vi "GDSLvIcon_AnalyseViIcon(ClassFix).vi"(0 "Class Ref":refnum<vi>, 1 "Class Private Data Control VI Ref":refnum<vi>, 3 "DoATextOCR(False)":bool, 5 "error in (no error)":errorcluster) -> (6 "BodyTextColor":u32(colorbox), 7 "Splitter0px":bool, 8 "HeaderTextColor":u32(colorbox), 9 "BodyText(OCR)":string, 10 "FrameColor":u32(colorbox), 11 "HeadText(OCR)":string, 12 "FrameThickness(1)":u32=1, 13 "ValidHeaderIcon":bool, 14 "DefaultIcon":bool, 15 "HeaderIcon":u8[][](array[numeric]) format="%x", 16 "HeaderBkColor":u32(colorbox), 17 "BodyIcon":u8[][](array[numeric]) format="%x", 18 "BodyBkColor":u32(colorbox), 19 "error out":errorcluster)   [LabVIEW 2020]
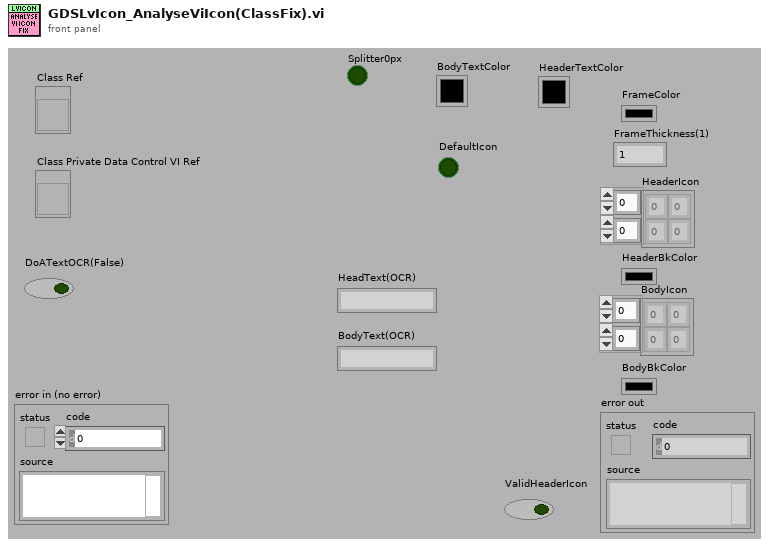
[diagram p1: front panel]
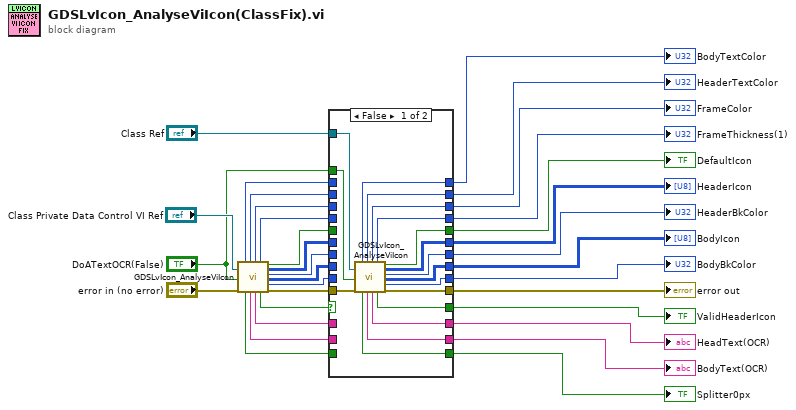
[diagram p0: block diagram]
diagram:
  n1 = call <resource>:"GDSLvIcon_AnalyseViIcon.vi"("ViRef/LvCLassRef/LvLibRef/ViPath/2D_Image"="Class Private Data Control VI Ref", "DoATextOCR(False)"="DoATextOCR(False)", "error in (no error)"="error in (no error)") -> ("BodyTextColor"=w10:u32, "Splitter0px"=w28:bool, "HeaderTextColor"=w12:u32, "BodyText(OCR)"=w27:string, "FrameColor"=w14:u32, "HeadText(OCR)"=w26:string, "FrameThickness(1)"=w16:u32, "ValidHeaderIcon"=w31:bool, "DefaultIcon"=w17:bool, "HeaderIcon"=w22:u8[][], "HeaderBkColor"=w24:u32, "BodyIcon"=w23:u8[][], "BodyBkColor"=w25:u32, "error out"=w5:errorcluster)  [unwired: 3 in]
  n2 = case shown="False" w31 {
    selector: w31 -> [_ w50]
    tunnel: "Class Ref" -> [w49 _]
    tunnel: w28 -> [_ w53]
    tunnel: w27 -> [_ w54]
    tunnel: w26 -> [_ w55]
    tunnel: w25 -> [_ w51]
    tunnel: w24 -> [_ w61]
    tunnel: [w37 w63] -> w20
    tunnel: w23 -> [_ w63]
    tunnel: [w39 w62] -> w21
    tunnel: w22 -> [_ w62]
    tunnel: [w38 w61] -> w19
    tunnel: [w40 w60] -> w18
    tunnel: w17 -> [_ w60]
    tunnel: w16 -> [_ w59]
    tunnel: [w41 w59] -> w15
    tunnel: w14 -> [_ w58]
    tunnel: [w42 w58] -> w13
    tunnel: w12 -> [_ w57]
    tunnel: [w43 w57] -> w11
    tunnel: w10 -> [_ w56]
    tunnel: [w44 w56] -> w9
    tunnel: [w34 w55] -> w8
    tunnel: [w33 w54] -> w7
    tunnel: [w46 w53] -> w6
    tunnel: w5 -> [w48 w52]
    tunnel: [w47 w52] -> w4
    tunnel: "DoATextOCR(False)" -> [w45 _]
    tunnel: [w36 w51] -> w1
    tunnel: [w35 w50] -> w2
    frame False {
      n3 = call <resource>:"GDSLvIcon_AnalyseViIcon.vi"("ViRef/LvCLassRef/LvLibRef/ViPath/2D_Image"=w49, "DoATextOCR(False)"=w45, "error in (no error)"=w48) -> ("BodyTextColor"=w44:u32, "Splitter0px"=w46:bool, "HeaderTextColor"=w43:u32, "BodyText(OCR)"=w33:string, "FrameColor"=w42:u32, "HeadText(OCR)"=w34:string, "FrameThickness(1)"=w41:u32, "ValidHeaderIcon"=w35:bool, "DefaultIcon"=w40:bool, "HeaderIcon"=w39:u8[][], "HeaderBkColor"=w38:u32, "BodyIcon"=w37:u8[][], "BodyBkColor"=w36:u32, "error out"=w47:errorcluster)  [unwired: 3 in]
    }
    frame True {
    }
  }
  "error out" <- w4
  "FrameColor" <- w13
  "BodyIcon" <- w20
  "HeaderIcon" <- w21
  "FrameThickness(1)" <- w15
  "HeaderBkColor" <- w19
  "BodyBkColor" <- w1
  "ValidHeaderIcon" <- w2
  "HeaderTextColor" <- w11
  "BodyTextColor" <- w9
  "BodyText(OCR)" <- w7
  "HeadText(OCR)" <- w8
  "DefaultIcon" <- w18
  "Splitter0px" <- w6
